vi "getPackageLicense.vi"(8 "error":errorcluster, 10 "pckg":string, 11 "connection ID":refnum<k5>) -> (0 "error out":errorcluster, 2 "string":string, 3 "connection ID out":refnum<k5>)   [LabVIEW 2016, in "amc_api.lvlib"]
doc: "Gets the license for a specific package."
uses:
  amc_api.lvlib
panel:
  out "jsonRespIn":string
  out "JSON-response":string="{\"jsonrpc\":\"2.0\",\"method\":\"\",\"params\":[5,1.245,true,\"name\"],\"id\":\"1\"}"
  out "JSON request":string
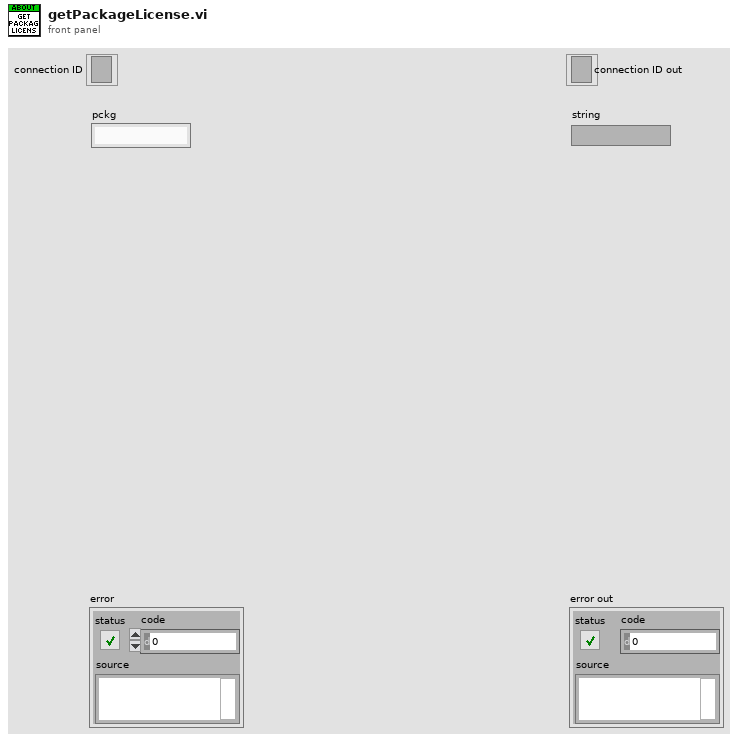
[diagram p1: front panel]
types:
  T1 = cluster{"jsonrpc":string, "method":string, "params":string[], "id":string, "api":i32, "pid":string}
  T2 = enum16{"Standard", "Buffered", "CRLF", "Immediate"}
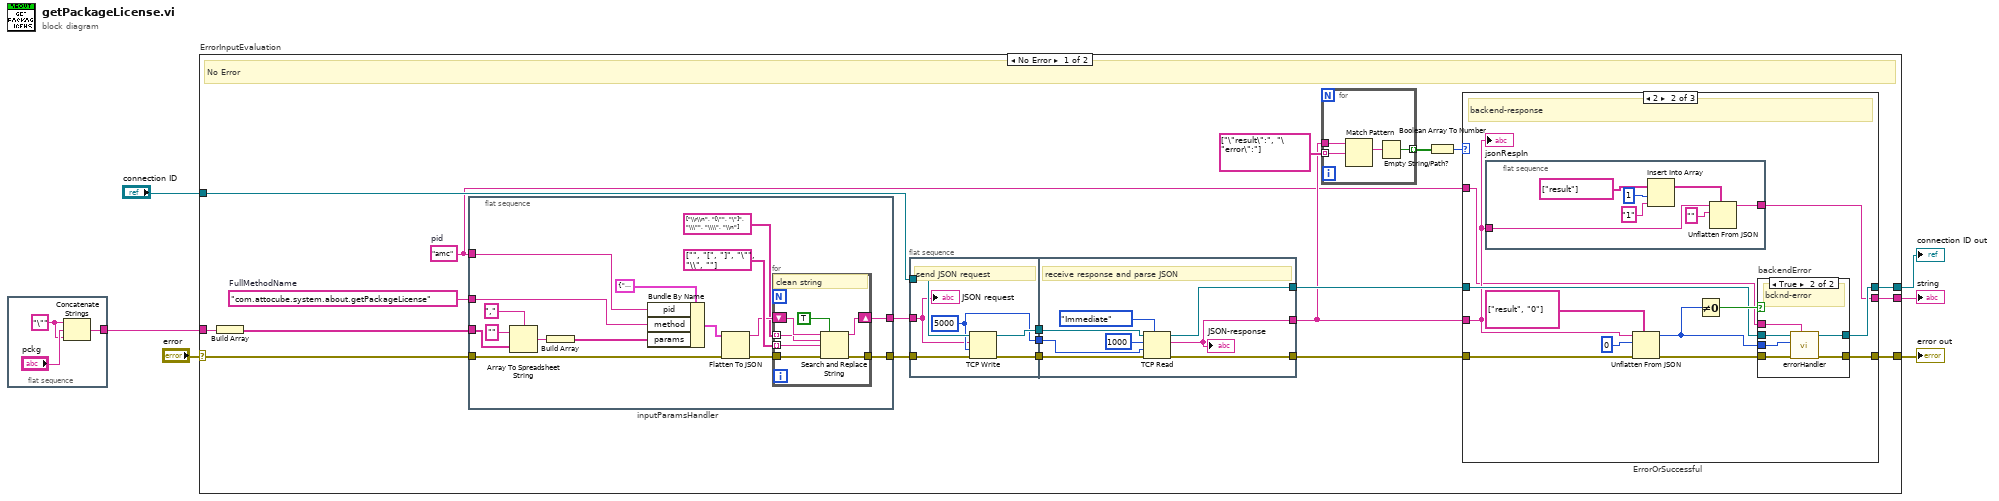
[diagram p0: block diagram]
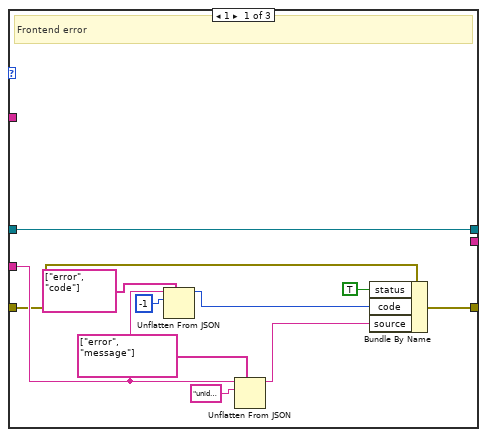
[diagram p2: hidden frame]
diagram:
  n1 = flat-sequence "in_string" {
    tunnel: [w8] -> w2
    frame #0 {
      w7 = "\"" ("string")
      n2 = Concatenate Strings(w7, "pckg", w7) -> (w8:string)
    }
  }
  n3 = case "ErrorInputEvaluation" shown="No Error" "error" {
    selector: "error" -> [w16 w111]
    tunnel: "connection ID" -> [w26 w112]
    tunnel: [w18 w111] -> w5
    tunnel: [w19 w112] -> w4
    tunnel: w2 -> [w11 _]
    tunnel: [w10 _] -> w1
    frame No Error {
      w12 = "amc"  # pid
      w17 = "com.attocube.system.about.getPackageLicense"  # FullMethodName
      # "No Error"
      n4 = Build Array ("ParametersArrayString")(w11) -> (w15:string[])
      n5 = flat-sequence "inputParamsHandler" {
        tunnel: [w35] -> w14
        tunnel: w15 -> [w41]
        tunnel: w16 -> [w40]
        tunnel: [w37] -> w13
        tunnel: w17 -> [w31]
        tunnel: w12 -> [w30]
        frame #0 {
          n6 = Array To Spreadsheet String(delimiter (Tab)=",", array=w41, 3:"" ("format string")) -> (spreadsheet string=w43:string)
          n7 = Build Array "Build Array"(w43) -> (w32:string[])
          n8 = Bundle By Name(cluster=T1 {"jsonrpc"="2.0", "method"="com.attocube.amc.res.setRESReadOutFreq", "params"=[], "id"="1", "api"=2, "pid"=""}, "pid"=w30, "method"=w31, "params"=w32) -> (w42:T1)
          n9 = Flatten To JSON(anything=w42, error in (no error)=w40) -> (JSON string=w36:string, 11:w38:errorcluster)  [unwired: 1 in]
          n10 = for {
            tunnel: string[] ["\\r\\n", "[\"", "\"]", "\\\"", "\\\\", "\\n"] ("search string") -> [w49] mode=indexing
            tunnel: string[] ["", "[", "]", "\"", "\\", ""] ("replace string (\"\")") -> [w48] mode=indexing
            shift-right: [w51] -> w35
            shift-left: w36 -> [w50]
            tunnel: w38 -> [w47]
            tunnel: [w46] -> w37
            # "clean string"
            n11 = Search and Replace String(replace all?=TRUE ("replace all? (F)"), input string=w50, search string=w49, replace string=w48, error in=w47) -> (result string=w51:string, error out=w46:errorcluster)  [unwired: 3 in, 2 out]
          }
        }
      }
      n12 = flat-sequence {
        tunnel: w26 -> [w102]
        tunnel: [w100] -> w29
        tunnel: [w101] -> w28
        tunnel: w13 -> [w97]
        tunnel: [w99] -> w27
        tunnel: w14 -> [w98]
        tunnel: [w106] -> w22
        tunnel: w29 -> [w108]
        tunnel: w28 -> [w107]
        tunnel: [w104] -> w21
        tunnel: w27 -> [w105]
        tunnel: [w103] -> w20
        frame #0 {
          w99 = 5000 ("timeout ms (25000)")
          # "send JSON request"
          n13 = TCP Write(connection ID=w102, data in=w98, error in (no error)=w97, 9:w99) -> (connection ID out=w100:refnum<k5>, error out=w101:errorcluster)  [unwired: 1 out]
          "JSON request" <- w98
        }
        frame #1 {
          # "receive response and parse JSON"
          n14 = TCP Read(connection ID=w108, bytes to read=1000, error in (no error)=w107, 7:T2."Immediate" ("mode (standard)"), 9:w105) -> (connection ID out=w106:refnum<k5>, data out=w103:string, error out=w104:errorcluster)
          "JSON-response" <- w103
        }
      }
      n15 = for {
        tunnel: string[] ["\"result\":", "\"error\":"] ("path") -> [w55] mode=indexing
        tunnel: [w53] -> w24 mode=indexing
        tunnel: w20 -> [w56]
        n16 = Match Pattern(string=w56, regular expression=w55) -> (match substring=w54:string)  [unwired: 1 in, 3 out]
        n17 = Empty String/Path?(string/path=w54) -> (empty?=w53:bool)
      }
      n18 = Boolean Array To Number(Boolean array=w24) -> (number=w23:u32)
      n19 = case "ErrorOrSuccessful" shown="2" w23 {
        tunnel: w20 -> [w59 w70 _]
        tunnel: w22 -> [w57 w73 w96]
        tunnel: [w57 w72 w96] -> w19
        tunnel: [w60 w71 w95] -> w18
        tunnel: w21 -> [w58 w74 w95]
        tunnel: w12 -> [_ w69 _]
        tunnel: [_ w68 _] -> w10
        frame 1 {
          # "Frontend error"
          n20 = Unflatten From JSON(path=string[] ["error", "code"], JSON string=w59, type and defaults=-1) -> (value=w66:i32)  [unwired: 4 in, 1 out]
          n21 = Unflatten From JSON(path=string[] ["error", "message"], JSON string=w59, type and defaults="unidentified error") -> (value=w67:string)  [unwired: 4 in, 1 out]
          n22 = Bundle By Name(cluster=w58, "status"=TRUE, "code"=w66, "source"=w67) -> (w60:errorcluster)
        }
        frame 2 {
          # "backend-response"
          n23 = flat-sequence "out_string" {
            tunnel: w70 -> [w86]
            tunnel: [w80] -> w68
            frame #0 {
              n24 = Insert Into Array(array=string[] ["result"] ("path"), index=1, new element="1" ("idx")) -> (w83:string[])
              n25 = Unflatten From JSON(path=w83, JSON string=w86, type and defaults="") -> (value=w80:string)  [unwired: 4 in, 1 out]
            }
          }
          n26 = Unflatten From JSON(path=string[] ["result", "0"], JSON string=w70, type and defaults=0, error in (no error)=w74) -> (value=w79:i32, error out=w77:errorcluster)  [unwired: 3 in]
          n27 = Not Equal To 0?(x=w79) -> (x != 0?=w78:bool)
          n28 = case "backendError" shown="True" w78 {
            tunnel: w79 -> [_ w94]
            tunnel: w77 -> [w88 w93]
            tunnel: [w87 w92] -> w72
            tunnel: [w88 w91] -> w71
            tunnel: w73 -> [w87 w90]
            tunnel: w69 -> [_ w89]
            frame False {
              # "successful"
            }
            frame True {
              # "bcknd-error"
              n29 = call "errorHandler.vi"("pid"=w89, "error in"=w93, "errNbr"=w94, "connection ID"=w90) -> ("error out 2"=w91:errorcluster, "connection ID out"=w92:refnum<k5>)  [unwired: 6 in]
            }
          }
          "jsonRespIn" <- w70
        }
        frame Default {
          # "NoResponse"
        }
      }
    }
    frame Error {
      # "Error"
    }
  }
  "error out" <- w5
  "connection ID out" <- w4
  "string" <- w1
